vi "subVI_CONEX_incrMove.vi"(0 "CONEX Cluster":T1, 1 "Motors to move":bool[](array[boolean]), 2 "Incr. Move (um default)":dbl[](array[numeric]), 3 "Error IN":errorcluster, 4 "Units":enum16{"mm", "um", "nm"}(ring)) -> (6 "CONEX Cluster out":T1, 9 "error out":errorcluster)   [LabVIEW 2010]
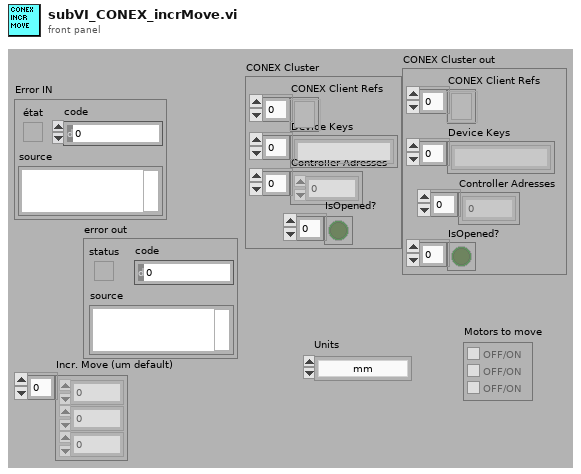
[diagram p1: front panel]
types:
  T1 = cluster{"CONEX Client Refs":refnum<k24>[], "Device Keys":string[], "Controller Adresses":i32[], "IsOpened?":bool[]}
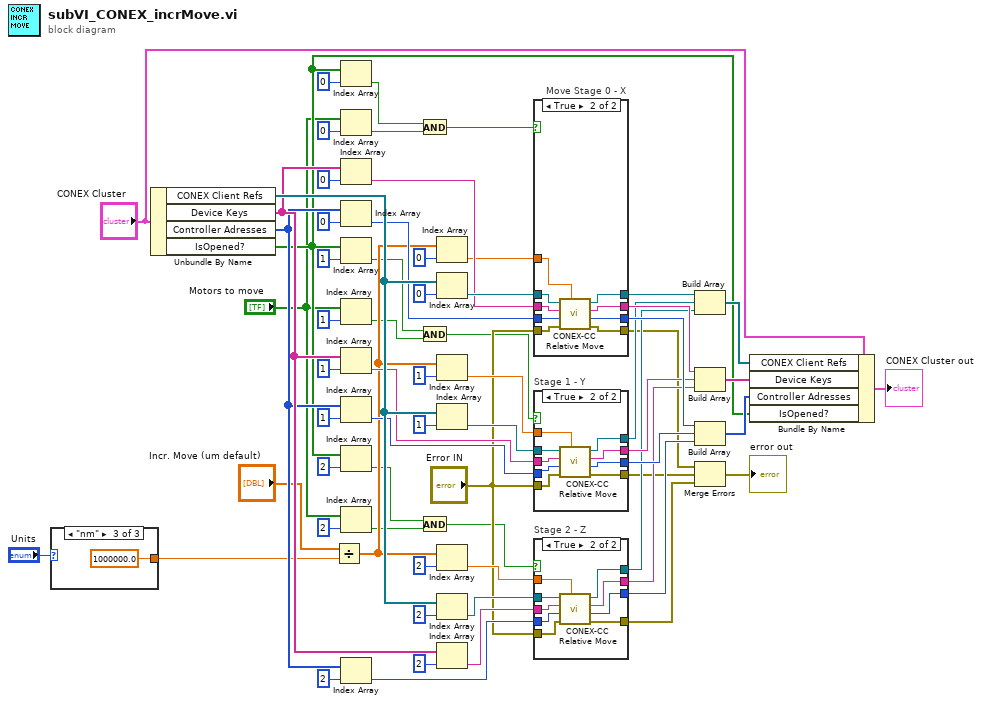
[diagram p0: block diagram]
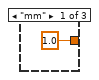
[diagram p2: hidden frame]
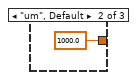
[diagram p3: hidden frame]
diagram:
  n1 = case shown="\"nm\"" "Units" {
    tunnel: [1.0 1000.0 1000000.0] -> w15
    frame "mm" {
    }
    frame "um", Default {
    }
    frame "nm" {
    }
  }
  n2 = Unbundle By Name("CONEX Cluster") -> ("CONEX Client Refs"=w64:refnum<k24>[], "Device Keys"=w59:string[], "Controller Adresses"=w54:i32[], "IsOpened?"=w19:bool[])
  n3 = Divide(x="Incr. Move (um default)", y=w15) -> (x/y=w14:dbl[])
  n4 = Index Array(array=w19, index=0) -> (element=w9:bool)
  n5 = Index Array(array="Motors to move", index=0) -> (element=w3:bool)
  n6 = Index Array(array=w59, index=0) -> (element=w58:string)
  n7 = Index Array(array=w54, index=0) -> (element=w53:i32)
  n8 = Index Array(array=w19, index=1) -> (element=w11:bool)
  n9 = Index Array(array="Motors to move", index=1) -> (element=w2:bool)
  n10 = Index Array(array=w59, index=1) -> (element=w35:string)
  n11 = Index Array(array=w54, index=1) -> (element=w32:i32)
  n12 = Index Array(array=w19, index=2) -> (element=w13:bool)
  n13 = Index Array(array="Motors to move", index=2) -> (element=w1:bool)
  n14 = Index Array(array=w54, index=2) -> (element=w33:i32)
  n15 = And(x=w9, y=w3) -> (x .and. y?=w8:bool)
  n16 = And(x=w11, y=w2) -> (x .and. y?=w10:bool)
  n17 = And(x=w13, y=w1) -> (x .and. y?=w12:bool)
  n18 = Index Array(array=w14, index=0) -> (element=w43:dbl)
  n19 = Index Array(array=w64, index=0) -> (element=w63:refnum<k24>)
  n20 = Index Array(array=w14, index=1) -> (element=w39:dbl)
  n21 = Index Array(array=w64, index=1) -> (element=w38:refnum<k24>)
  n22 = Index Array(array=w14, index=2) -> (element=w36:dbl)
  n23 = Index Array(array=w64, index=2) -> (element=w37:refnum<k24>)
  n24 = Index Array(array=w59, index=2) -> (element=w34:string)
  n25 = case "Move Stage 0 - X" shown="True" w8 {
    tunnel: w63 -> [w71 w83]
    tunnel: w58 -> [w72 w82]
    tunnel: w53 -> [w73 w81]
    tunnel: "Error IN" -> [w74 w80]
    tunnel: [w71 w79] -> w52
    tunnel: [w72 w78] -> w51
    tunnel: [w73 w77] -> w50
    tunnel: w43 -> [_ w76]
    tunnel: [w74 w75] -> w21
    frame False {
    }
    frame True {
      n26 = call <userlib>:"CONEX-CC Relative Move.vi"("Relative displacement"=w76, "Error IN"=w80, "Address IN"=w81, "deviceKey IN"=w82, "CONEX Client Ref IN"=w83) -> ("Error OUT"=w75:errorcluster, "Address OUT"=w77:i32, "deviceKey OUT"=w78:string, "CONEX Client Ref OUT"=w79:refnum<k24>)  [unwired: 1 in]
    }
  }
  n27 = case "Stage 1 - Y" shown="True" w10 {
    tunnel: w38 -> [w84 w96]
    tunnel: w35 -> [w85 w95]
    tunnel: w32 -> [w86 w94]
    tunnel: "Error IN" -> [w87 w93]
    tunnel: [w84 w92] -> w25
    tunnel: [w85 w91] -> w28
    tunnel: [w86 w90] -> w29
    tunnel: w39 -> [_ w89]
    tunnel: [w87 w88] -> w24
    frame False {
    }
    frame True {
      n28 = call <userlib>:"CONEX-CC Relative Move.vi"("Relative displacement"=w89, "Error IN"=w93, "Address IN"=w94, "deviceKey IN"=w95, "CONEX Client Ref IN"=w96) -> ("Error OUT"=w88:errorcluster, "Address OUT"=w90:i32, "deviceKey OUT"=w91:string, "CONEX Client Ref OUT"=w92:refnum<k24>)  [unwired: 1 in]
    }
  }
  n29 = case "Stage 2 - Z" shown="True" w12 {
    tunnel: w37 -> [w97 w109]
    tunnel: w34 -> [w98 w108]
    tunnel: w33 -> [w99 w107]
    tunnel: "Error IN" -> [w100 w106]
    tunnel: [w97 w105] -> w26
    tunnel: [w98 w104] -> w27
    tunnel: [w99 w103] -> w30
    tunnel: w36 -> [_ w102]
    tunnel: [w100 w101] -> w23
    frame False {
    }
    frame True {
      n30 = call <userlib>:"CONEX-CC Relative Move.vi"("Relative displacement"=w102, "Error IN"=w106, "Address IN"=w107, "deviceKey IN"=w108, "CONEX Client Ref IN"=w109) -> ("Error OUT"=w101:errorcluster, "Address OUT"=w103:i32, "deviceKey OUT"=w104:string, "CONEX Client Ref OUT"=w105:refnum<k24>)  [unwired: 1 in]
    }
  }
  n31 = Build Array(w52, w25, w26) -> (w49:refnum<k24>[])
  n32 = Build Array(w51, w28, w27) -> (w48:string[])
  n33 = Build Array(w50, w29, w30) -> (w47:i32[])
  n34 = Merge Errors(w21, w24, w23) -> (→"error out":errorcluster)
  n35 = Bundle By Name(cluster="CONEX Cluster", "CONEX Client Refs"=w49, "Device Keys"=w48, "Controller Adresses"=w47, "IsOpened?"=w19) -> (→"CONEX Cluster out":T1)
